vi "UndoButtonWasPressed.vi"(8 "error in (no error)":errorcluster, 11 "reference in":refnum<class "RemoteControl.lvclass">) -> (0 "error out":errorcluster, 3 "reference out":refnum<class "RemoteControl.lvclass">)   [LabVIEW 2020, in "RemoteControl.lvclass"]
uses:
  RemoteControl.lvclass
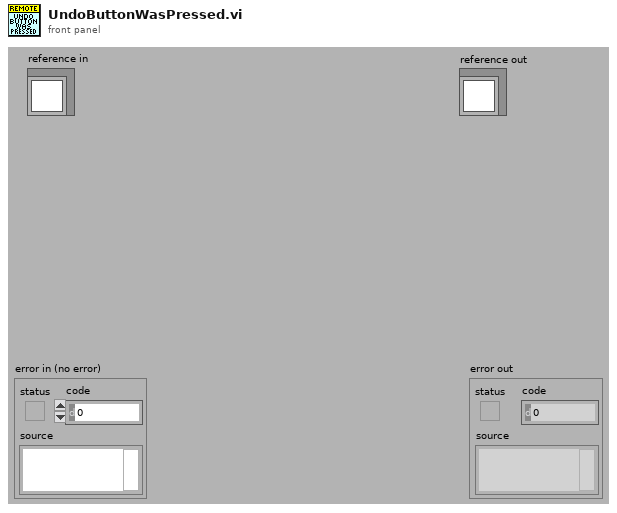
[diagram p1: front panel]
types:
  T1 = typedef "RemoteControl.lvclass/ObjectAttributes.ctl" = cluster{"OnCommands":refnum<class "Command.lvclass">[], "OffCommands":refnum<class "Command.lvclass">[], "UndoCommand":refnum<class "Command.lvclass">}
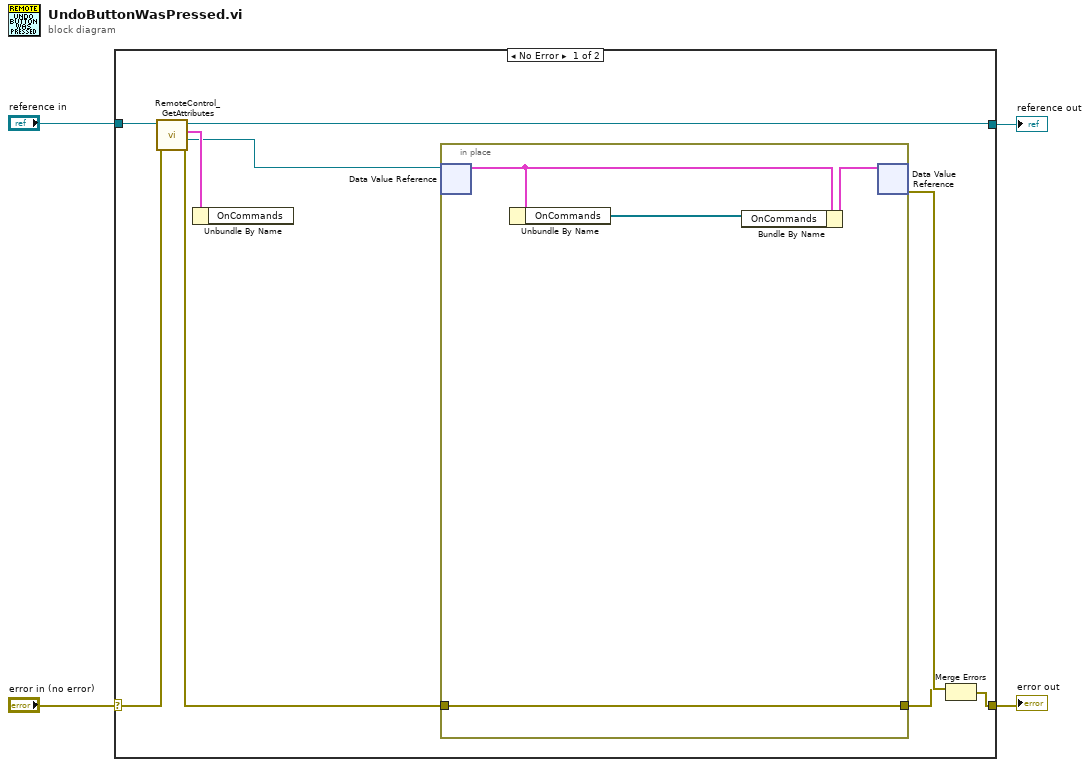
[diagram p0: block diagram]
diagram:
  n1 = case shown="No Error" "error in (no error)" {
    selector: "error in (no error)" -> [w12 w19]
    tunnel: [w8 w19] -> w3
    tunnel: [w9 w18] -> w1
    tunnel: "reference in" -> [w13 w18]
    frame No Error {
      n2 = call "RemoteControl_GetAttributes.vi"("error in (no error)"=w12, "reference in"=w13) -> ("error out"=w6:errorcluster, "DataRef"=w7:refnum<data-value>, "Data"=w11:T1, "reference out"=w9:refnum<class "RemoteControl.lvclass">)  [unwired: 6 in]
      n3 = Unbundle By Name(w11) -> ()  [unwired: 1 out]
      n4 = in-place {
        in-place-border: w6 -> [w16]
        in-place-border: [w16] -> w5
        n5 = in-place-dvr #1(w7) -> (w15:T1)  [unwired: 1 out]
        n6 = Unbundle By Name(w15) -> ("OnCommands"=w14:refnum<class "Command.lvclass">[])
        n7 = Bundle By Name(cluster=w15, "OnCommands"=w14) -> (w17:T1)
        n8 = in-place-dvr #1(w17) -> (w10:errorcluster)  [unwired: 1 out]
      }
      n9 = Merge Errors(w10, w5) -> (w8:errorcluster)
    }
    frame Error {
    }
  }
  "error out" <- w3
  "reference out" <- w1
